vi "conMem.vi"(3 "error in":errorcluster, 4 "Memory":T1, 5 "InstrumentID":u32) -> (0 "error out":errorcluster, 1 "Status":i32 format="%.0x")   [LabVIEW 2022 SP3]
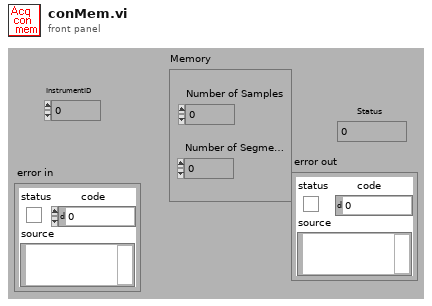
[diagram p1: front panel]
types:
  T1 = cluster{"Number of Samples":i32, "Number of Segments":i32}
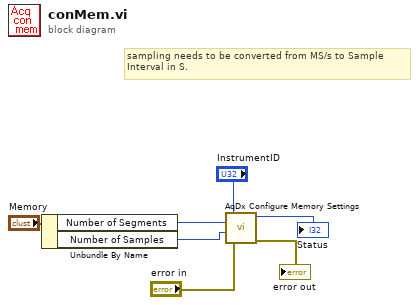
[diagram p0: block diagram]
diagram:
  # "sampling needs to be converted from MS/s to Sample\nInterval in S."
  n1 = Unbundle By Name("Memory") -> ("Number of Segments"=w3:i32, "Number of Samples"=w4:i32)
  n2 = call "AqDx Configure Memory Settings.vi"("error in (no error)"="error in", "Number of Samples (1000)"=w4, "Number of Segments (1)"=w3, "Instrument ID"="InstrumentID") -> ("error out"=→"error out":errorcluster, "dup Instrument ID"=→"Status":u32)  [unwired: 2 in]
